vi "magnet ramp to field vector.vi"(4 "const phi?":bool, 6 "Delta H (mT)":dbl=0.5 format="%.3f", 7 "error in (no error)":errorcluster, 8 "sweep parameter":T1=enum."magnetic field", 9 "delta phi (deg)":dbl=0.5, 10 "magnet polar":T3 {"theta" format="%#_3g"; "phi" format="%#_3g"; "magnitude" format="%#_3g"}) -> (0 "error out":errorcluster, 3 "Current Magnetic\nField\n(430 TCP reading)":T2 {"phi (deg)" format="%#_4f"})   [LabVIEW 2013]
uses:
  magnet polar field.ctl
  AMI reading polar field.ctl
  measurement/measurement sweep parameter.ctl
  app/app global state actions.ctl
  config.vi
panel:
  # "! BEFORE EXECUTING, MAKE SURE SWITCH HTRS ARE ON\nby running magnet initialize.vi !"
  # "Negative magnitude leads to angle inversion"
  # "Delta phi applies only for angle sweep and is always >0! \nIt is the angle increment size during angle sweep to achieve rotation at constant magnitude. Suggestion: 0.5 deg. Make sure it is a multiple of your sweep increment during the measurement. E.g. record spectra for 1, 2, 3 deg rather than 1.2, 2.2, 3.2 deg. if delta phi is 0.5deg.\nAlso, you cannot perform angle sweeps with less than 1deg. step."
  # "Theta is set by the motor."
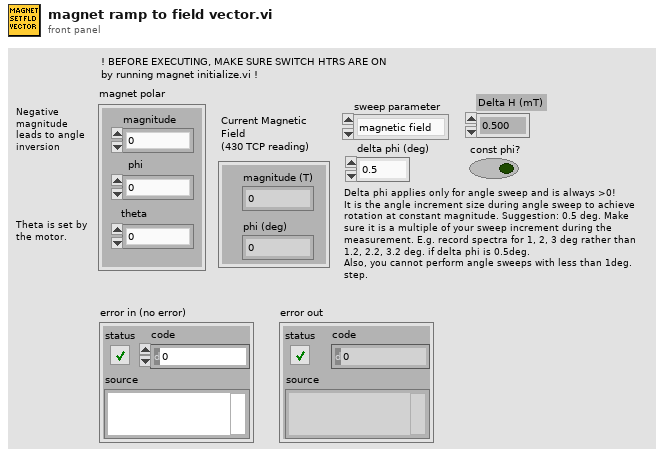
[diagram p1: front panel]
types:
  T1 = typedef "measurement sweep parameter.ctl" = enum16{"angle", "magnetic field"}
  T2 = typedef "AMI reading polar field.ctl" = cluster{"magnitude (T)":dbl, "phi (deg)":dbl}
  T3 = typedef "magnet polar field.ctl" = cluster{"magnitude":dbl, "phi":dbl, "theta":dbl}
  T4 = typedef "app global state actions.ctl" = enum16{"set field reached", "get cluster", "set cluster", "set current sweep", "set field value", "set 430 TCP reading", "set ramping", "set sweeping", "append log", "clear log", "set finished"}
  T5 = cluster{"GPIB address":i16, "GPIB bus":i16, "connection ID":refnum<k5>, "IP":string, "Active Comm Interface":u16, "Serial Port":refnum<visa-resource-name>, "Programmer Type":u16}
  T6 = cluster{"error":bool, "code":i32, "source":string}
  T7 = typedef "app global state control.ctl" = cluster{"current field value":T3, "field ramping":bool, "vna sweeping":bool, "Log Messages":string, "current sweep":T8, "measurement finished":bool, "Current Magnetic Field\n(430 TCP reading)":cluster{"magnitude (T)":dbl, "phi (deg)":dbl}, "field was reached":bool}
  T8 = typedef "measconfig cluster.ctl" = cluster{"sweep parameter":T1, "sweep start":dbl, "sweep stop":dbl, "sweep increment":dbl, "temperature":dbl, "path":path, "magnet initial":T3, "magnet reference":T3, "const phi?":bool, "delta phi (deg)":dbl, "delta H (mT)":dbl, "const phi init field?":bool}
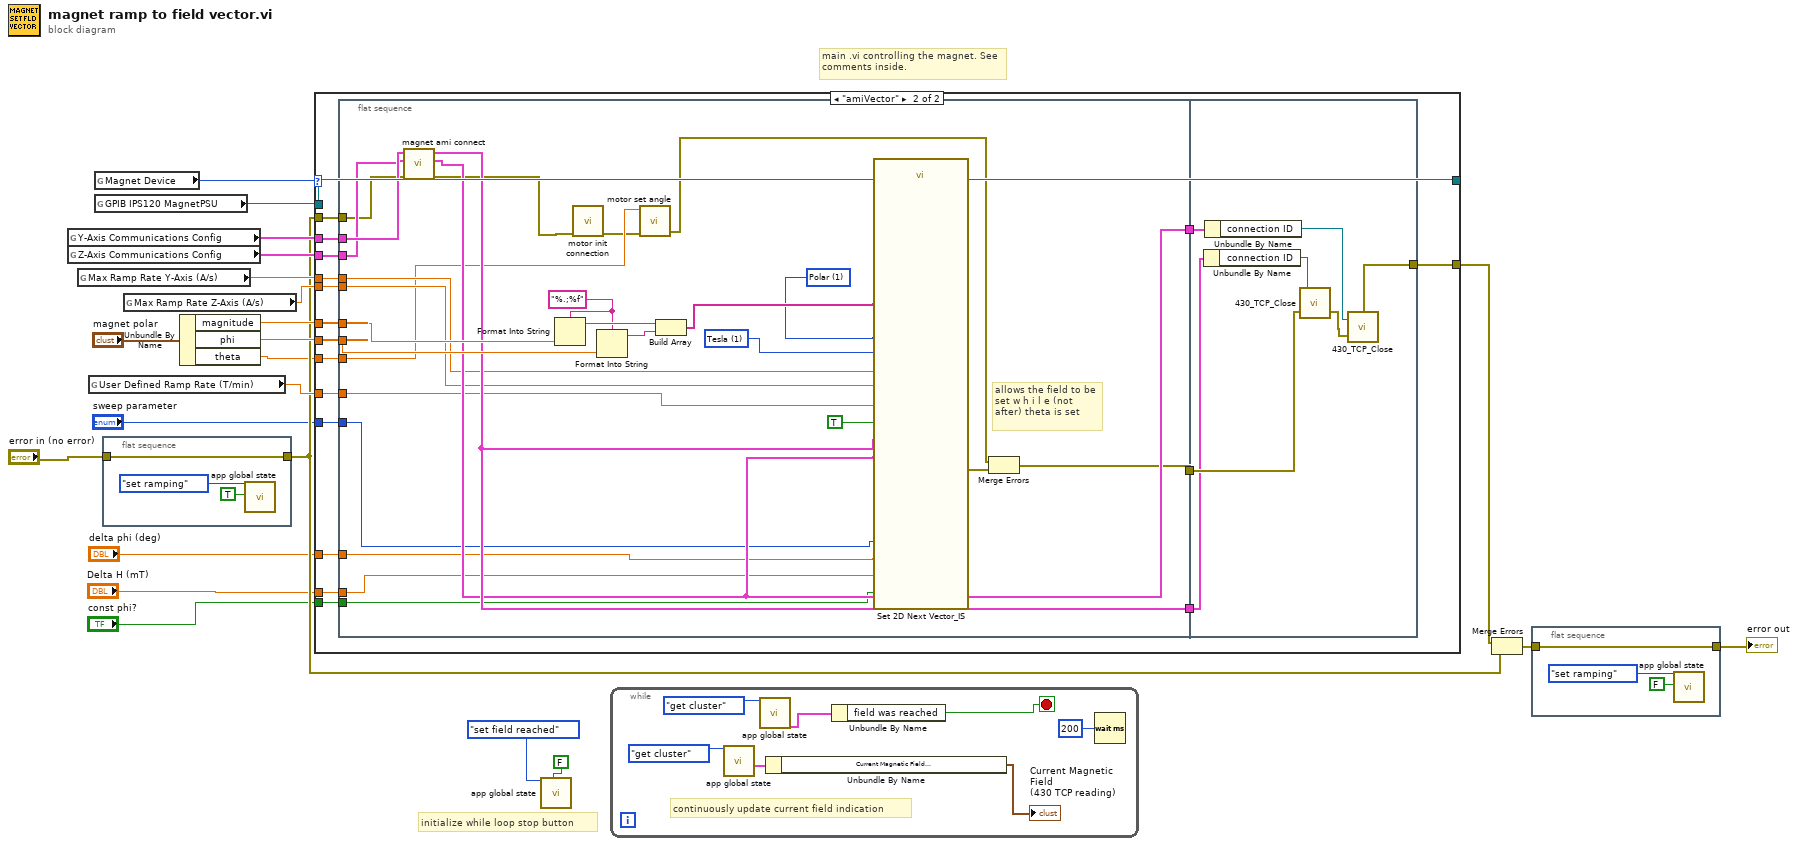
[diagram p0: block diagram]
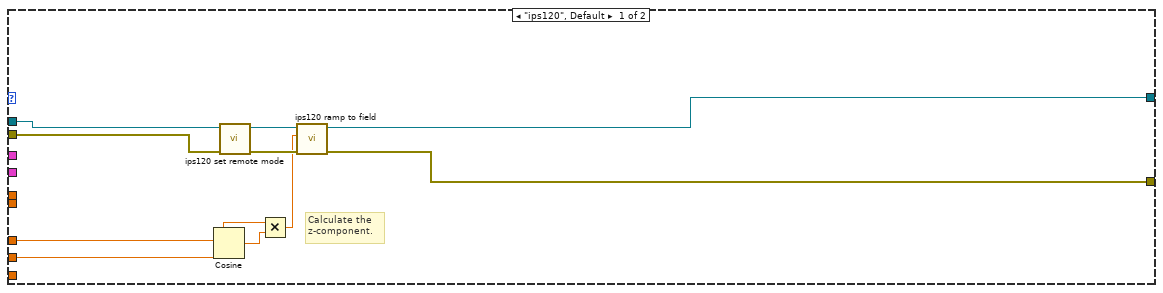
[diagram p2: hidden frame]
diagram:
  # "main .vi controlling the magnet. See comments inside."
  # "initialize while loop stop button"
  n1 = global read "config.vi" "Y-Axis Communications Config"() -> (w19:T5)
  n2 = global read "config.vi" "Z-Axis Communications Config"() -> (w18:T5)
  n3 = global read "config.vi" "Max Ramp Rate Y-Axis (A/s)"() -> (w11:dbl)
  n4 = global read "config.vi" "User Defined Ramp Rate (T/min)"() -> (w9:dbl)
  n5 = global read "config.vi" "Magnet Device"() -> (w21:enum16{"ips120", "amiVector"})
  n6 = global read "config.vi" "GPIB IPS120 MagnetPSU"() -> (w20:refnum<visa-resource-name>)
  n7 = flat-sequence {
    tunnel: "error in (no error)" -> [w25]
    tunnel: [w25] -> w8
    frame #0 {
      n8 = call "app global state.vi"("action"=app_global_state_actions."set ramping" ("app global state actions"), "field ramping"=TRUE) -> ()  [unwired: 17 in, 1 out]
    }
  }
  n9 = global read "config.vi" "Max Ramp Rate Z-Axis (A/s)"() -> (w10:dbl)
  n10 = Unbundle By Name("magnet polar") -> ("magnitude"=w16:dbl, "phi"=w17:dbl, "theta"=w1:dbl)
  n11 = case shown="\"amiVector\"" w21 {
    tunnel: w20 -> [w29 w53]
    tunnel: w19 -> [_ w52]
    tunnel: w18 -> [_ w51]
    tunnel: w17 -> [w35 w47]
    tunnel: w16 -> [w34 w48]
    tunnel: w8 -> [w32 w50]
    tunnel: [w30 w49] -> w15
    tunnel: [w27 w53] -> _
    tunnel: w11 -> [_ w44]
    tunnel: w10 -> [_ w45]
    tunnel: w9 -> [_ w46]
    tunnel: "sweep parameter" -> [_ w40]
    tunnel: "delta phi (deg)" -> [_ w39]
    tunnel: "Delta H (mT)" -> [_ w38]
    tunnel: "const phi?" -> [_ w37]
    tunnel: w1 -> [_ w36]
    frame "ips120", Default {
      # "Calculate the \nz-component."
      n12 = Cosine(x=w35) -> (cos(x)=w33:dbl)
      n13 = call "ips120 set remote mode.vi"("error in (no error)"=w32, "VISA resource name"=w29) -> ("error out"=w31:errorcluster, "VISA resource name 2"=w28:refnum<visa-resource-name>)  [unwired: 8 in]
      n14 = Multiply(x=w34, y=w33) -> (x*y=w26:dbl)
      n15 = call "ips120 ramp to field.vi"("error in (no error)"=w31, "target field (T)"=w26, "VISA resource name"=w28) -> ("error out"=w30:errorcluster, "VISA resource name 2"=w27:refnum<visa-resource-name>)  [unwired: 7 in]
    }
    frame "amiVector" {
      n16 = flat-sequence {
        tunnel: w52 -> [w77]
        tunnel: w51 -> [w76]
        tunnel: w50 -> [w60]
        tunnel: w48 -> [w75]
        tunnel: w47 -> [w74]
        tunnel: w46 -> [w63]
        tunnel: w45 -> [w61]
        tunnel: w44 -> [w62]
        tunnel: [w56] -> w43
        tunnel: [w69] -> w42
        tunnel: [w70] -> w41
        tunnel: w40 -> [w68]
        tunnel: w39 -> [w67]
        tunnel: w38 -> [w66]
        tunnel: w37 -> [w65]
        tunnel: w36 -> [w59]
        tunnel: [w87] -> w49
        tunnel: w43 -> [w85]
        tunnel: w42 -> [w82]
        tunnel: w41 -> [w81]
        frame #0 {
          w78 = "%.;%f" ("format string")
          w72 = u16 1 items=["Cartesian", "Polar"] ("Coordinate System")
          w71 = u16 1 items=["kG", "Tesla"] ("Magnetic Field Units")
          # "allows the field to be set w h i l e (not after) theta is set"
          n17 = call "magnet ami connect.vi"("error in (no error)"=w60, "Z-Axis Communications Config"=w76, "Y-Axis Communications Config"=w77) -> ("error out"=w57:errorcluster, "Z-Axis Communications Config Out"=w69:T5, "Y-Axis Communications Config Out"=w70:T5)  [unwired: 6 in]
          n18 = Format Into String(format string=w78, w75) -> (resulting string=w80:string)  [unwired: 2 in, 1 out]
          n19 = call "motor init connection.vi"("error in (no error)"=w57) -> ("error out"=w58:errorcluster)  [unwired: 9 in, 1 out]
          n20 = Format Into String(format string=w78, w74) -> (resulting string=w79:string)  [unwired: 2 in, 1 out]
          n21 = call "motor set angle.vi"("error in (no error)"=w58, "angle"=w59) -> ("error out"=w54:errorcluster)  [unwired: 9 in]
          n22 = Build Array(w80, w79) -> (w73:string[])
          n23 = call "Set 2D Next Vector_IS.vi"("Coordinate System"=w72, "Magnetic Field Units"=w71, "Input Vector"=w73, "User defined Ramp Rate (T/min)"=w63, "Y-Axis Communications Config"=w70, "sweep parameter"=w68, "Z-Axis Communications Config"=w69, "Delta phi (deg)"=w67, "Delta H (mT)"=w66, "User defined Ramp Rate?"=TRUE ("User defined Ramp Rate (T/min)"), "Max Ramp Rate - Y Axis (A/s)"=w62, "const phi?"=w65, "Max Ramp Rate - Z Axis (A/s)"=w61) -> ("error out"=w55:T6)  [unwired: 9 in, 5 out]
          n24 = Merge Errors(w54, w55) -> (w56:errorcluster)
        }
        frame #1 {
          n25 = Unbundle By Name(w81) -> ("connection ID"=w83:refnum<k5>)
          n26 = Unbundle By Name(w82) -> ("connection ID"=w84:refnum<k5>)
          n27 = call <userlib>:"430_TCP_Close.vi"("error in (no error)"=w85, "connection ID"=w83) -> ("error out"=w86:errorcluster)  [unwired: 1 out]
          n28 = call <userlib>:"430_TCP_Close.vi"("error in (no error)"=w86, "connection ID"=w84) -> ("error out"=w87:errorcluster)  [unwired: 1 out]
        }
      }
    }
  }
  n29 = call "app global state.vi"("action"=app_global_state_actions."set field reached" ("app global state actions"), "field was reached"=FALSE ("measurement finished")) -> ()  [unwired: 17 in, 1 out]
  n30 = while {
    stop <- w91 stop-if-true
    # "continuously update current field indication"
    n31 = call "app global state.vi"("action"=app_global_state_actions."get cluster" ("app global state actions")) -> ("global state"=w89:T7)  [unwired: 18 in]
    n32 = call "app global state.vi"("action"=app_global_state_actions."get cluster" ("app global state actions")) -> ("global state"=w93:T7)  [unwired: 18 in]
    n33 = Unbundle By Name(w89) -> ("Current Magnetic Field\n(430 TCP reading)"=→"Current Magnetic\nField\n(430 TCP reading)":cluster{"magnitude (T)":dbl, "phi (deg)":dbl})
    n34 = Unbundle By Name(w93) -> ("field was reached"=w91:bool)
    n35 = Wait (ms)(milliseconds to wait=200) -> ()  [unwired: 1 out]
  }
  n36 = Merge Errors(w15, w8) -> (w13:errorcluster)
  n37 = flat-sequence {
    tunnel: w13 -> [w97]
    tunnel: [w97] -> w12
    frame #0 {
      n38 = call "app global state.vi"("action"=app_global_state_actions."set ramping" ("app global state actions"), "field ramping"=FALSE) -> ()  [unwired: 17 in, 1 out]
    }
  }
  "error out" <- w12
